vi "ASIC_CONFIGURAR SALIDAS LVDS ENA.vi"(7 "Espera acceso USB":u32=10, 8 "error in":errorcluster, 9 "LVDS ENA 1":bool, 10 "LVDS ENA 0":bool, 11 "ftHandle_in":u32) -> (0 "error out":errorcluster, 3 "ftHandle_out":u32)   [LabVIEW 2019]
panel:
  out "test":u16 format="%04x"
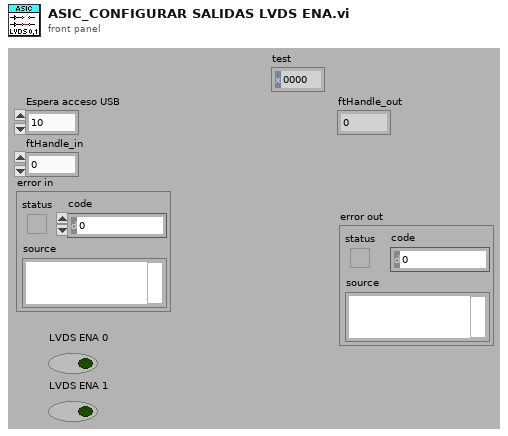
[diagram p1: front panel]
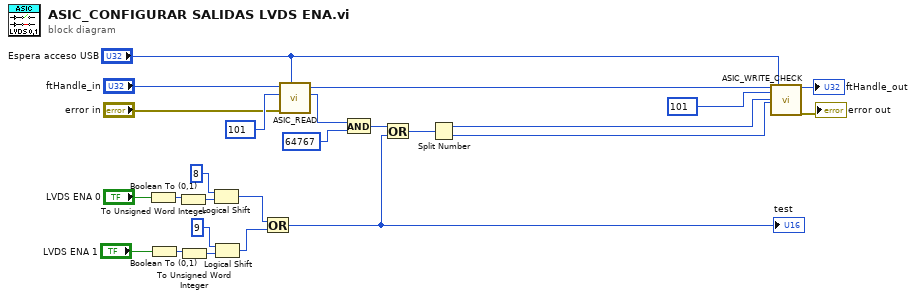
[diagram p0: block diagram]
diagram:
  n1 = Boolean To (0,1)(Boolean="LVDS ENA 0") -> (0, 1=w4:i16)
  n2 = Boolean To (0,1)(Boolean="LVDS ENA 1") -> (0, 1=w9:i16)
  n3 = To Unsigned Word Integer(number=w4) -> (unsigned 16bit integer=w3:u16)
  n4 = To Unsigned Word Integer(number=w9) -> (unsigned 16bit integer=w10:u16)
  n5 = Logical Shift(y=u16 8 ("x"), x=w3) -> (x << y=w2:u16)
  n6 = Logical Shift(y=u16 9 ("x"), x=w10) -> (x << y=w7:u16)
  n7 = Or(x=w2, y=w7) -> (x .or. y?=w6:u16)
  "test" <- w6
  n8 = call "ASIC_READ.vi"("Espera acceso USB"="Espera acceso USB", "error in"="error in", "Direccion Registro Asic"=u8 101, "ftHandle_in"="ftHandle_in") -> ("Valor Asic"=w15:u16, "ftHandle_out"=w18:u32)  [unwired: 5 in, 1 out]
  n9 = And(x=w15, y=u16 64767) -> (x .and. y?=w13:u16)
  n10 = Or(x=w13, y=w6) -> (x .or. y?=w12:u16)
  n11 = Split Number(x=w12) -> (hi(x)=w17:u8, lo(x)=w16:u8)
  n12 = call "ASIC_WRITE_CHECK.vi"("ftHandle_in"=w18, "Direccion Registro Asic"=u8 101, "Byte Alto"=w17, "Byte Bajo"=w16, "Espera acceso USB 2"="Espera acceso USB") -> ("ftHandle_out"=→"ftHandle_out":u32, "error out"=→"error out":errorcluster)  [unwired: 12 in, 1 out]
